vi "Generate File Header.vi"(11 "Header Data":T1={"Operator Name"="John Doe", "UUT Serial Number"="A001", "Test Name"="Temperature"}) -> (3 "File Header":string)   [LabVIEW 2014]
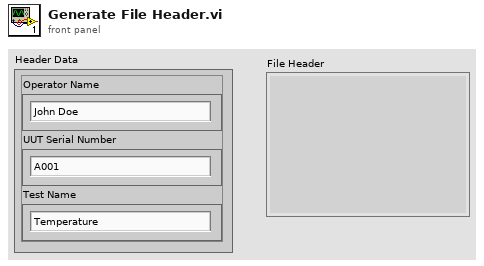
[diagram p1: front panel]
types:
  T1 = cluster{"Operator Name":string, "UUT Serial Number":string, "Test Name":string}
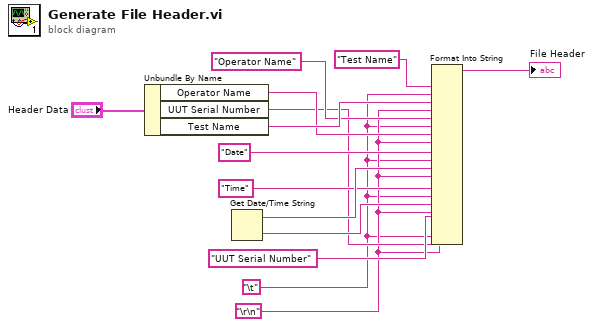
[diagram p0: block diagram]
diagram:
  w4 = "\r\n"
  w3 = "\t"
  n1 = Unbundle By Name("Header Data") -> ("Operator Name"=w11:string, "UUT Serial Number"=w5:string, "Test Name"=w13:string)
  n2 = Get Date/Time String() -> (date string=w9:string, time string=w7:string)  [unwired: 3 in]
  n3 = Format Into String("Test Name", w3, w13, w4, "Operator Name", w3, w11, w4, "Date", w3, w9, w4, "Time", w3, w7, w4, "UUT Serial Number", w3, w5, w4) -> (resulting string=→"File Header":string)  [unwired: 3 in, 1 out]
